vi "After Initialize.vi"(6 "State In":variant, 7 "Compiled Inline Async Settings":variant, 8 "error in":errorcluster, 9 "Custom Settings":variant, 10 "Compiled Settings":variant, 11 "CDAPI in":refnum<class "CustomDeviceAPI.lvclass">) -> (0 "error out":errorcluster, 3 "CDAPI out":refnum<class "CustomDeviceAPI.lvclass">, 4 "State Out":variant)   [LabVIEW 2026, in "Template Debug Tools.lvlib"]
uses:
  Template Debug Tools.lvlib
  <userlib>/CustomDeviceInterfaces_v1.lvlibp/custom-device-express-framework/Source/Custom Device Interfaces/CustomDeviceAPI/CustomDeviceAPI.lvclass
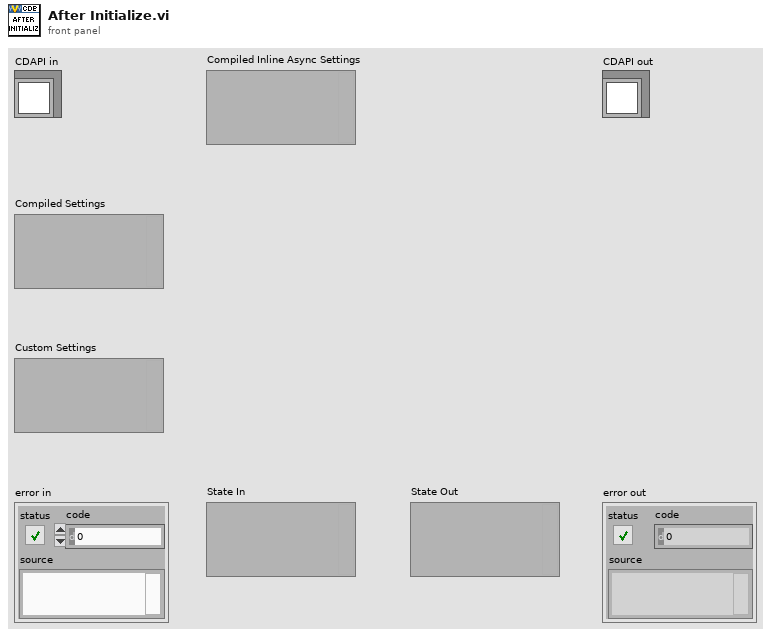
[diagram p1: front panel]
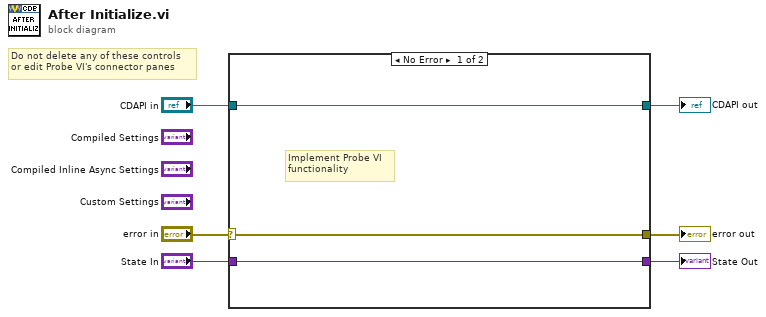
[diagram p0: block diagram]
diagram:
  # "Do not delete any of these controls\nor edit Probe VI's connector panes"
  n1 = case shown="No Error" "error in" {
    selector: "error in" -> [w9 w11]
    tunnel: [w9 w11] -> w5
    tunnel: "CDAPI in" -> [w8 w12]
    tunnel: [w8 w12] -> w3
    tunnel: "State In" -> [w7 w10]
    tunnel: [w7 w10] -> w1
    frame No Error {
      # "Implement Probe VI\nfunctionality"
    }
    frame Error {
    }
  }
  "CDAPI out" <- w3
  "error out" <- w5
  "State Out" <- w1
